vi "StartImageAcquisition.vi"(8 "error in (no error)":errorcluster, 11 "session in":T1) -> (0 "error out":errorcluster, 3 "session out":T1)   [LabVIEW 2017, in "IrAcquisition.lvlib"]
uses:
  <vilib>/addons/InsightCM/Devices/Shared/Ir/IrAcquisition/IrAcquisition.lvlib
  <vilib>/userdefined/High Color/IMAQdx.ctl
  <vilib>/vision/driver/NI_Vision_Acquisition_Software.lvlib
  <vilib>/vision/driver/IMAQdx.llb/IMAQdx Acquisition Mode.ctl
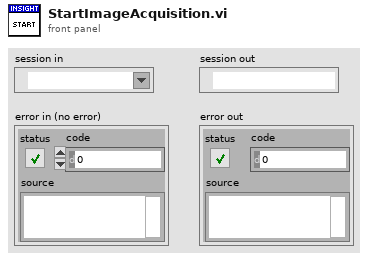
[diagram p1: front panel]
types:
  T1 = typedef "IMAQdx.ctl" = refnum<k21>
  T2 = typedef "NI_Vision_Acquisition_Software.lvlib/IMAQdx Acquisition Mode.ctl" = enum32{"One Shot", "Continuous"}
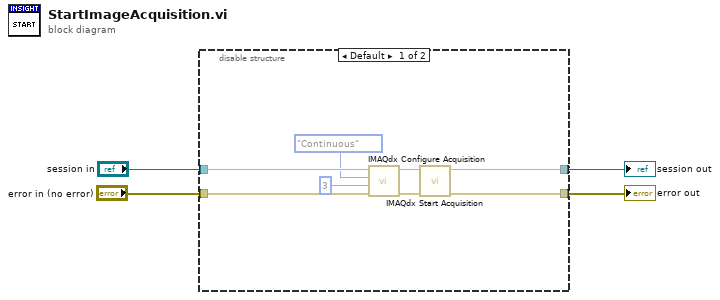
[diagram p0: block diagram]
diagram:
  n1 = disable-structure shown="Default" {
    disable-tunnel: [w12 w14] -> w4
    disable-tunnel: [w11 w13] -> w3
    disable-tunnel: "error in (no error)" -> [w10 w13]
    disable-tunnel: "session in" -> [w9 w14]
    frame condition #0 {
      n2 = call <vilib>:"IMAQdx Configure Acquisition.vi"("error in"=w10, "Number of Buffers"=u32 3, "Continuous?"=IMAQdx_Acquisition_Mode."Continuous", "Session In"=w9) -> ("error out"=w6:errorcluster, "Session Out"=w5:T1)  [unwired: 6 out]
      n3 = call <vilib>:"IMAQdx Start Acquisition.vi"("error in"=w6, "Session In"=w5) -> ("error out"=w11:errorcluster, "Session Out"=w12:T1)  [unwired: 8 out]
    }
    frame condition #1 (active) {
      # "simulated"
    }
  }
  "session out" <- w4
  "error out" <- w3
